vi "Ramsete_SINC.vi"(11 "IN VALUE":dbl) -> (3 "OUT SINC":dbl)   [LabVIEW 2019, in "Trajectory_Library.lvlib"]
doc: "Returns sin(x) / x\n\nWhen x is close to zero a special approximation calculation is used. Otherwise Sin(x)/X is used.\n\nParameters:\n - X - Input value"
uses:
  Trajectory_Library.lvlib
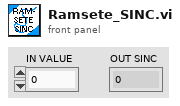
[diagram p1: front panel]
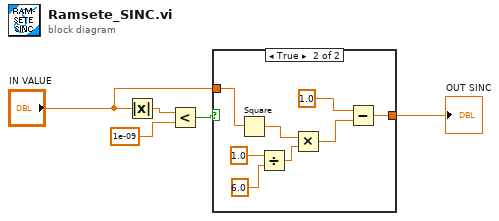
[diagram p0: block diagram]
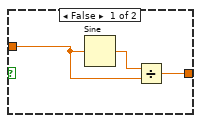
[diagram p2: hidden frame]
diagram:
  n1 = Absolute Value(x="IN VALUE") -> (abs(x)=w1:dbl)
  n2 = Less?(x=w1, y=1e-09) -> (x < y?=w3:bool)
  n3 = case shown="True" w3 {
    tunnel: "IN VALUE" -> [w7 w16]
    tunnel: [w6 w9] -> w4
    frame False {
      n4 = Sine(x=w7) -> (sin(x)=w8:dbl)
      n5 = Divide(x=w8, y=w7) -> (x/y=w6:dbl)
    }
    frame True {
      n6 = Square(x=w16) -> (x^2=w15:dbl)
      n7 = Divide(x=1.0, y=6.0) -> (x/y=w12:dbl)
      n8 = Multiply(x=w15, y=w12) -> (x*y=w11:dbl)
      n9 = Subtract(x=1.0, y=w11) -> (x-y=w9:dbl)
    }
  }
  "OUT SINC" <- w4
